vi "WFM Main.vi"() -> ()   [LabVIEW 2024]
doc: "Use this template to build a simple state machine design pattern. Each state executes code and determines which state to transition to."
uses:
  controls/WFM State.ctl
  controls/WFM Data.ctl
  controls/WFM Data Array.ctl
panel:
  out "Waveform Graph":dbl[](graph)
  in  "Log to File":bool
  in  "Acquire Waveform":bool
  in  "Exit":bool
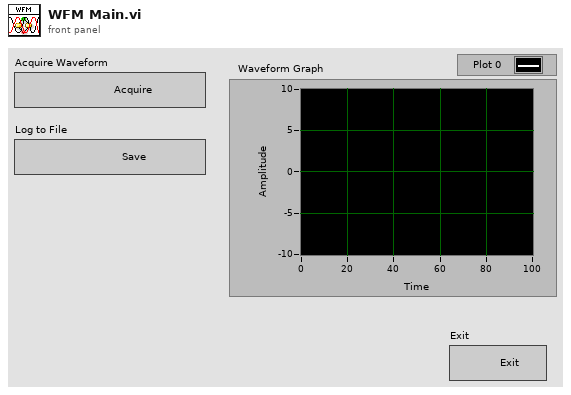
[diagram p1: front panel]
types:
  T1 = typedef "WFM Data.ctl" = cluster{"Array":T2[]}
  T2 = typedef "WFM Data Array.ctl" = dbl
  T3 = typedef "WFM State.ctl" = enum16{"Initialize", "Wait for Event", "Acquire Waveform", "Log to File", "Stop"}
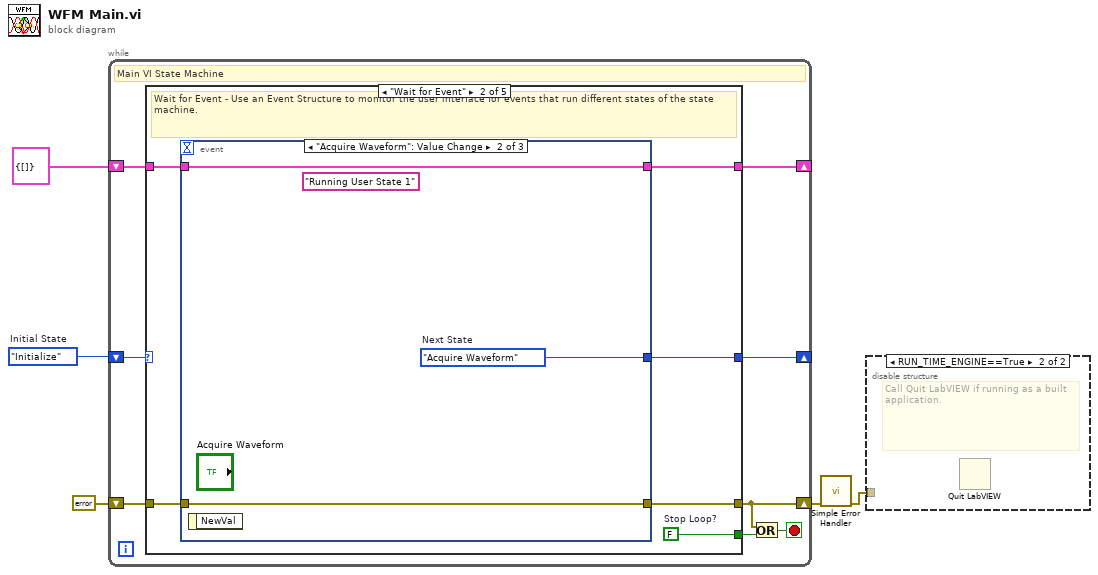
[diagram p0: block diagram]
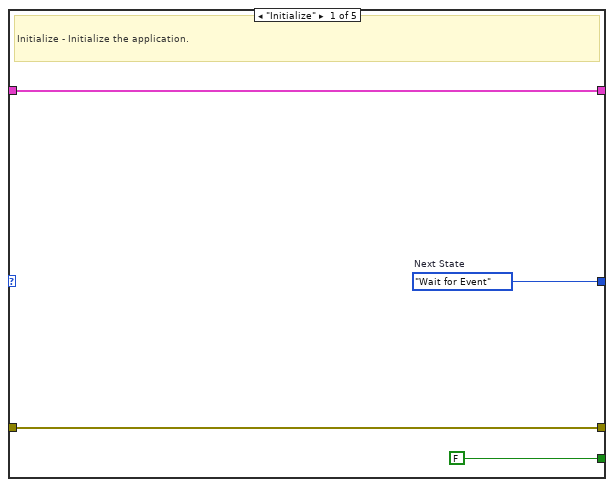
[diagram p3: hidden frame]
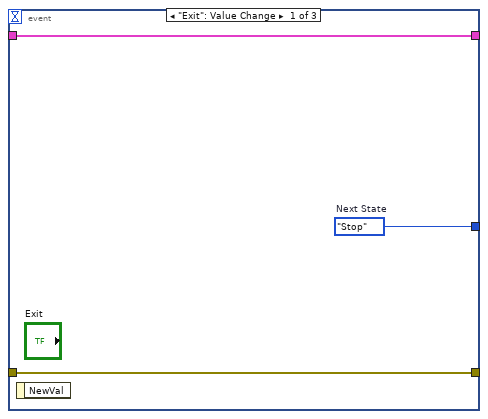
[diagram p4: hidden frame]
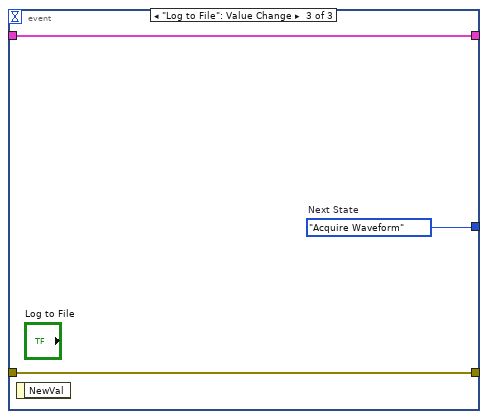
[diagram p5: hidden frame]
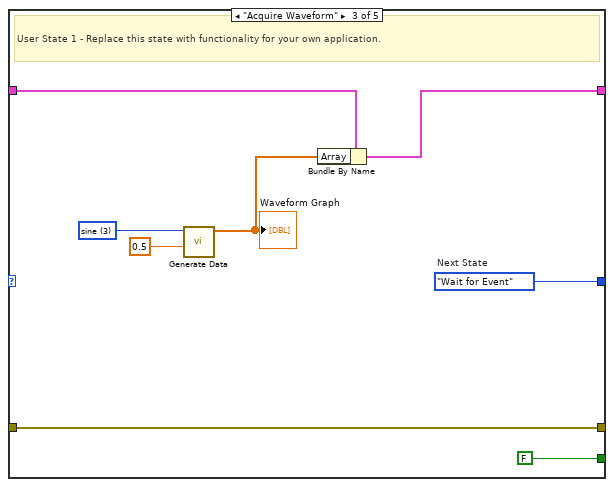
[diagram p6: hidden frame]
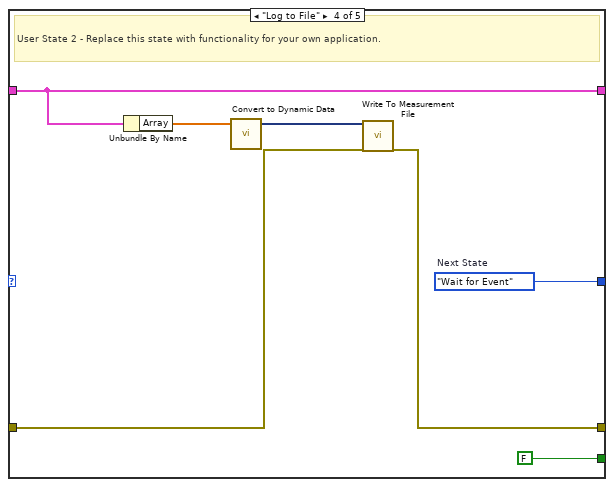
[diagram p7: hidden frame]
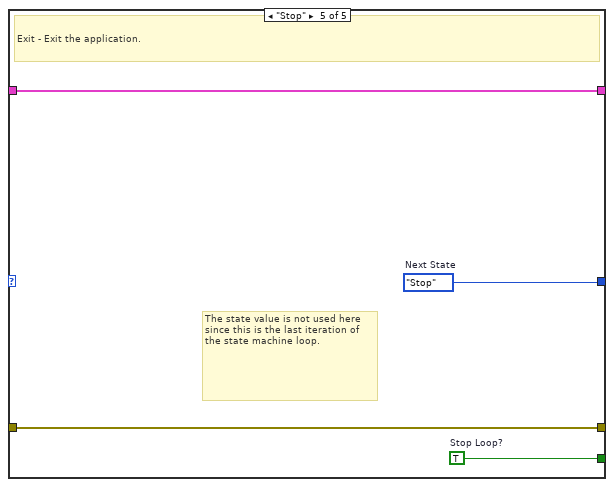
[diagram p8: hidden frame]
diagram:
  w5 = WFM_State."Initialize"  # Initial State
  n1 = while {
    shift-right: [w12] -> _
    shift-left: w5 -> [w13]
    shift-right: [w10] -> _
    shift-left: T1 {"Array"=[]} ("Data") -> [w11]
    shift-right: [w6] -> w2
    shift-left: errorcluster {"status"=FALSE, "code"=0, "source"=""} ("error constant") -> [w9]
    stop <- w7 stop-if-true
    # "Main VI State Machine"
    n2 = case shown="\"Wait for Event\"" w13 {
      tunnel: [w17 w23 w40 w47 w48] -> w12
      tunnel: [FALSE ("Stop Loop?") w22 FALSE ("Stop Loop?") FALSE ("Stop Loop?") w50] -> w8
      tunnel: w11 -> [w14 w21 w34 w45 w51]
      tunnel: [w14 w20 w33 w45 w51] -> w10
      tunnel: w9 -> [w15 w19 w38 w42 w49]
      tunnel: [w15 w18 w38 w41 w49] -> w6
      frame "Initialize" {
        w17 = WFM_State."Wait for Event"  # Next State
        # "Initialize - Initialize the application."
      }
      frame "Wait for Event" {
        w22 = FALSE  # Stop Loop?
        # "Wait for Event - Use an Event Structure to monitor the user interface for events that run different states of the state machine."
        n3 = event shown="[1] \"Acquire Waveform\": Value Change" {
          selector: _ -> [_ _ _]
          dyn-events: _ -> [_ _ _]
          timeout: _ -> [_ _ _]
          tunnel: [w24 w28 w31] -> w23
          tunnel: w21 -> [w26 w27 w30]
          tunnel: [w26 w27 w30] -> w20
          tunnel: w19 -> [w25 w29 w32]
          tunnel: [w25 w29 w32] -> w18
          event "Exit": Value Change {
            w24 = WFM_State."Stop"  # Next State
            n4 = event-data() -> ()  [unwired: 1 in, 1 out]
          }
          event "Acquire Waveform": Value Change {
            w28 = WFM_State."Acquire Waveform"  # Next State
            (unwired) "Running User State 1" ("Running User State 1")
            n5 = event-data() -> ()  [unwired: 1 in, 1 out]
          }
          event "Log to File": Value Change {
            w31 = WFM_State."Acquire Waveform"  # Next State
            n6 = event-data() -> ()  [unwired: 1 in, 1 out]
          }
        }
      }
      frame "Acquire Waveform" {
        w36 = u16 3 items=["uniform white", "uniform+uniform", "Gaussian white", "sine", "square"] ("signal")
        w40 = WFM_State."Wait for Event"  # Next State
        # "User State 1 - Replace this state with functionality for your own application."
        n7 = call "Generate Data.vi"("noise (rms)"=0.5, "signal"=w36) -> ("Y"=w37:dbl[])  [unwired: 8 in, 1 out]
        "Waveform Graph" <- w37
        n8 = Bundle By Name(cluster=w34, "Array"=w37) -> (w33:T1)
      }
      frame "Log to File" {
        w47 = WFM_State."Wait for Event"  # Next State
        # "User State 2 - Replace this state with functionality for your own application."
        n9 = Unbundle By Name "Unbundle By Name"(w45) -> ("Array"=w44:T2[])
        n10 = call "Convert to Dynamic Data"("Array"=w44) -> ("Dynamic Data Type"=w43:dynamicdata)  [unwired: 3 in]
        n11 = call "Write To Measurement File"("Signals"=w43, "error in (no error)"=w42) -> ("error out"=w41:errorcluster)  [unwired: 15 in, 2 out]
      }
      frame "Stop" {
        w48 = WFM_State."Stop"  # Next State
        w50 = TRUE  # Stop Loop?
        # "The state value is not used here since this is the last iteration of the state machine loop."
        # "Exit - Exit the application."
      }
    }
    n12 = Or(x=w6, y=w8) -> (x .or. y?=w7:bool)
  }
  n13 = call <vilib>:"Simple Error Handler.vi"("error in (no error)"=w2) -> ("error out"=w1:errorcluster)  [unwired: 4 in, 4 out]
  n14 = disable-structure shown="RUN_TIME_ENGINE==True" {
    disable-tunnel: w1 -> [_ _]
    frame condition #0 (active) {
    }
    frame condition #1 {
      # "Call Quit LabVIEW if running as a built application."
      n15 = Quit LabVIEW() -> ()  [unwired: 1 in]
    }
  }
